vi "ShowImage.vi"(11 "Image":T1 {"Dialogs" format="%.0b"}) -> (0 "picture":picture)   [LabVIEW 2013]
doc: "20feb20124 rjn: Created to convert image data to viewable picture"
uses:
  <vilib>/picture/picture.llb/Draw True-Color Pixmap.vi
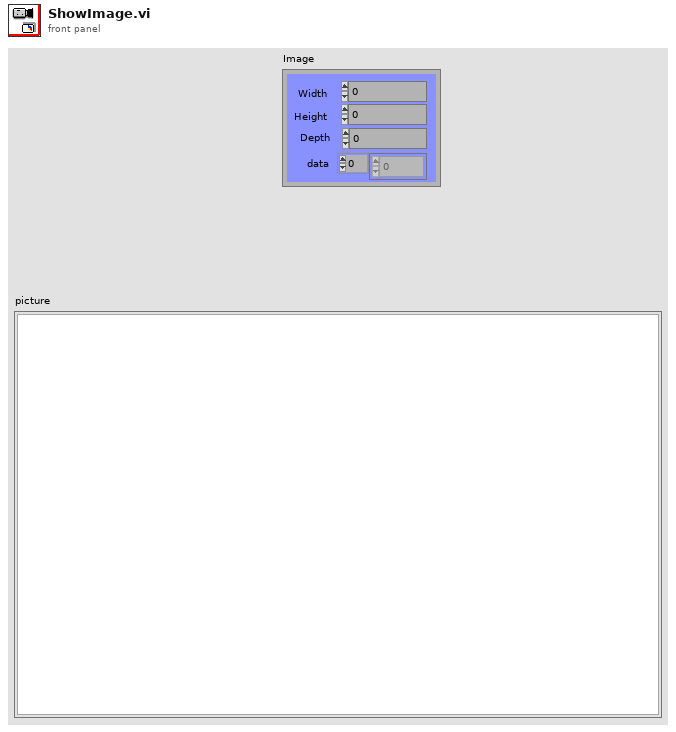
[diagram p1: front panel]
types:
  T1 = cluster{"Width":i32, "Height":i32, "Depth":i32, "data":u8[], "Compressed data":u8[], "Color table":u32[], "Duration":i32, "Options":i32, "Timestamp":i32, "ID":i32, "Reserved":i32, "Dialogs":u32}
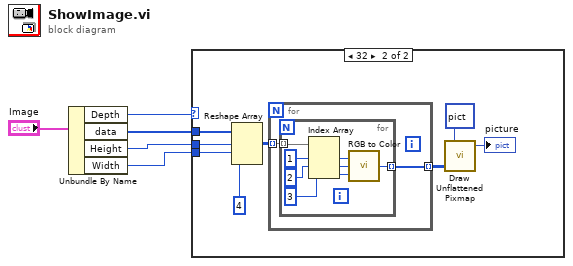
[diagram p0: block diagram]
diagram:
  n1 = Unbundle By Name("Image") -> ("Depth"=w4:i32, "data"=w3:u8[], "Height"=w2:i32, "Width"=w1:i32)
  n2 = case shown="32" w4 {
    tunnel: w2 -> [_ w8]
    tunnel: w3 -> [_ w7]
    tunnel: w1 -> [_ w6]
    frame 0, Default {
    }
    frame 32 {
      n3 = Reshape Array(w7, w8, w6, 4 ("dimension size")) -> (w10:u8[][][])
      n4 = for {
        tunnel: w10 -> [w15] mode=indexing
        tunnel: [w14] -> w13 mode=indexing
        n5 = for {
          tunnel: w15 -> [w17] mode=indexing
          tunnel: [w16] -> w14 mode=indexing
          n6 = Index Array(array=w17, index #1=1 ("index"), index #2=2 ("index"), index #3=3 ("index")) -> (element #1=w20:u8, element #2=w19:u8, element #3=w18:u8)
          n7 = call <vilib>:"RGB to Color.vi"("B"=w18, "G"=w19, "R"=w20) -> ("Color"=w16:u32)
        }
      }
      n8 = call-poly <vilib>:"Draw Unflattened Pixmap.vi"("picture"=picture data[5B], "data (RGB format)"=w13) -> ("new picture"=→"picture":picture)  [unwired: 7 in]
    }
  }
